vi "RP100SourVoltNow.vi"(3 "error in (no error)":errorcluster, 4 "Source":enum16{"1", "2"}(ring), 5 "VISA resource name":refnum<visa-resource-name>="COM8") -> (0 "error out":errorcluster, 1 "Voltage":dbl, 2 "VISA resource name out":refnum<visa-resource-name>)   [LabVIEW 2019, in "RP100.lvlib"]
uses:
  RP100.lvlib
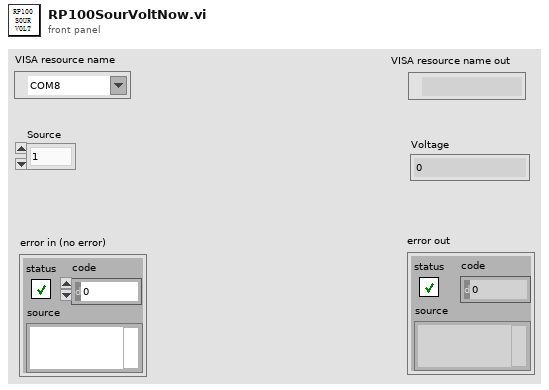
[diagram p1: front panel]
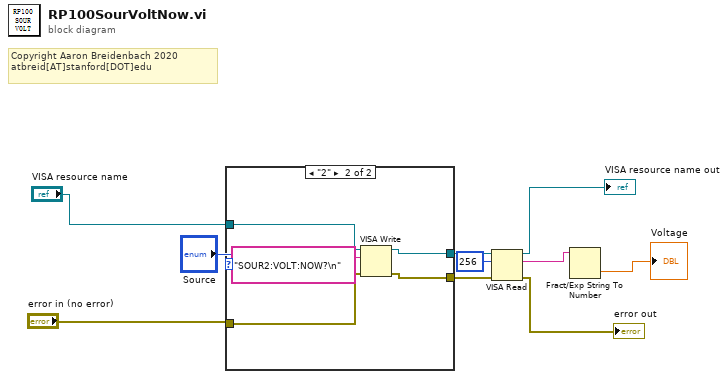
[diagram p0: block diagram]
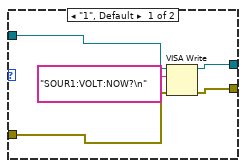
[diagram p2: hidden frame]
diagram:
  # "Copyright Aaron Breidenbach 2020\natbreid[AT]stanford[DOT]edu"
  n1 = case shown="\"2\"" "Source" {
    tunnel: "VISA resource name" -> [w14 w20]
    tunnel: "error in (no error)" -> [w13 w19]
    tunnel: [w12 w17] -> w9
    tunnel: [w11 w16] -> w8
    frame "1", Default {
      n2 = VISA Write(VISA resource name=w14, write buffer="SOUR1:VOLT:NOW?\n", error in (no error)=w13) -> (VISA resource name out=w12:refnum<visa-resource-name>, error out=w11:errorcluster)  [unwired: 1 out]
    }
    frame "2" {
      n3 = VISA Write(VISA resource name=w20, write buffer="SOUR2:VOLT:NOW?\n", error in (no error)=w19) -> (VISA resource name out=w17:refnum<visa-resource-name>, error out=w16:errorcluster)  [unwired: 1 out]
    }
  }
  n4 = VISA Read(VISA resource name=w9, byte count=u32 256, error in (no error)=w8) -> (VISA resource name out=→"VISA resource name out":refnum<visa-resource-name>, read buffer=w4:string, error out=→"error out":errorcluster)  [unwired: 1 out]
  n5 = Fract/Exp String To Number(string=w4) -> (number=→"Voltage":dbl)  [unwired: 3 in, 1 out]
